vi "set step rate.vi"(8 "error in":errorcluster, 9 "axis (def: fine)":enum16{"fine", "coarse"}(ring), 10 "step rate":dbl, 11 "GPIB # (in): def. 6":string="6") -> (0 "error out":errorcluster, 3 "GPIB # (out)":string)   [LabVIEW 2017]
uses:
  mc2mc4.llb/MC2/4  SendCommand.VI
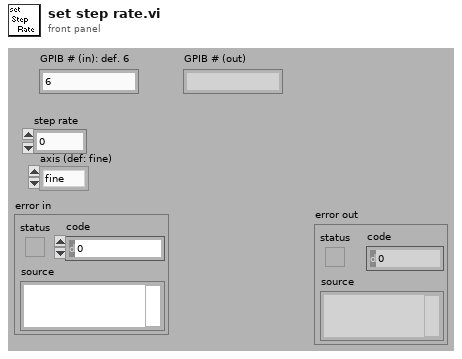
[diagram p1: front panel]
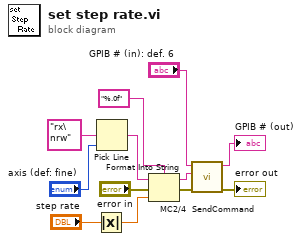
[diagram p0: block diagram]
diagram:
  n1 = Absolute Value(x="step rate") -> (abs(x)=w8:dbl)
  n2 = Pick Line(multi-line string="rx\nrw", line index="axis (def: fine)") -> (output string=w6:string)  [unwired: 1 out]
  n3 = Format Into String ("Set number of\n Big Steps")(format string="%.0f", initial string=w6, error in="error in", w8) -> (resulting string=w11:string, error out=w10:errorcluster)
  n4 = call "MC2/4  SendCommand.VI"("error in (no error)"=w10, "MC2 / MC4 Command"=w11, "GPIB # (in): def.6"="GPIB # (in): def. 6") -> ("error out"=→"error out":errorcluster, "GPIB # (out)"=→"GPIB # (out)":string)  [unwired: 7 out]
